vi "img test 4.vi"() -> ()   [LabVIEW 2009]
uses:
  <vilib>/vision/NI_Vision_Development_Module.lvlib
panel:
  in  "Number of Erosion":i32=2
  in  "Number of iterations (1) 3":i32=1
  in  "Structuring Element 3":i32[][](array[numeric])=[[1, 0, 0, 0, 0], [0, 0, 0, 0, 0], [0, 0, 0, 0, 0], [0, 0, 0, 0, 0], [0, 0, 0, 0, 1]]
  in  "Operation 3":T1(ring)=enum."Erode"
  out "appended array":cluster{"Numeric":dbl, "Numeric":dbl}[](array[cluster])
  out "Image 5":T2(plugin-control)
  in  "Number of iterations (1) 2":i32=1
  in  "Structuring Element 2":i32[][](array[numeric])=[[1, 0, 0, 0, 0], [0, 0, 0, 0, 0], [0, 0, 0, 0, 0], [0, 0, 0, 0, 0], [0, 0, 0, 0, 1]]
  in  "Operation 2":T1(ring)=enum."Erode"
  in  "Range 2":cluster{"Lower value":sgl, "Upper value":sgl}={"Lower value"=128.0, "Upper value"=255.0} {"Upper value" format="%.2f"; "Lower value" format="%.2f"}
  out "Image":T2(plugin-control)
  in  "stop":bool
  out "Image 2":T2(plugin-control)
  in  "frame diff":i32
  in  "startign rame":i32
  in  "AVI Path":path=path "C:/Users/Kokum Weeratunga/Desktop/ChongWei vs LinDan (japan open 2010).avi"
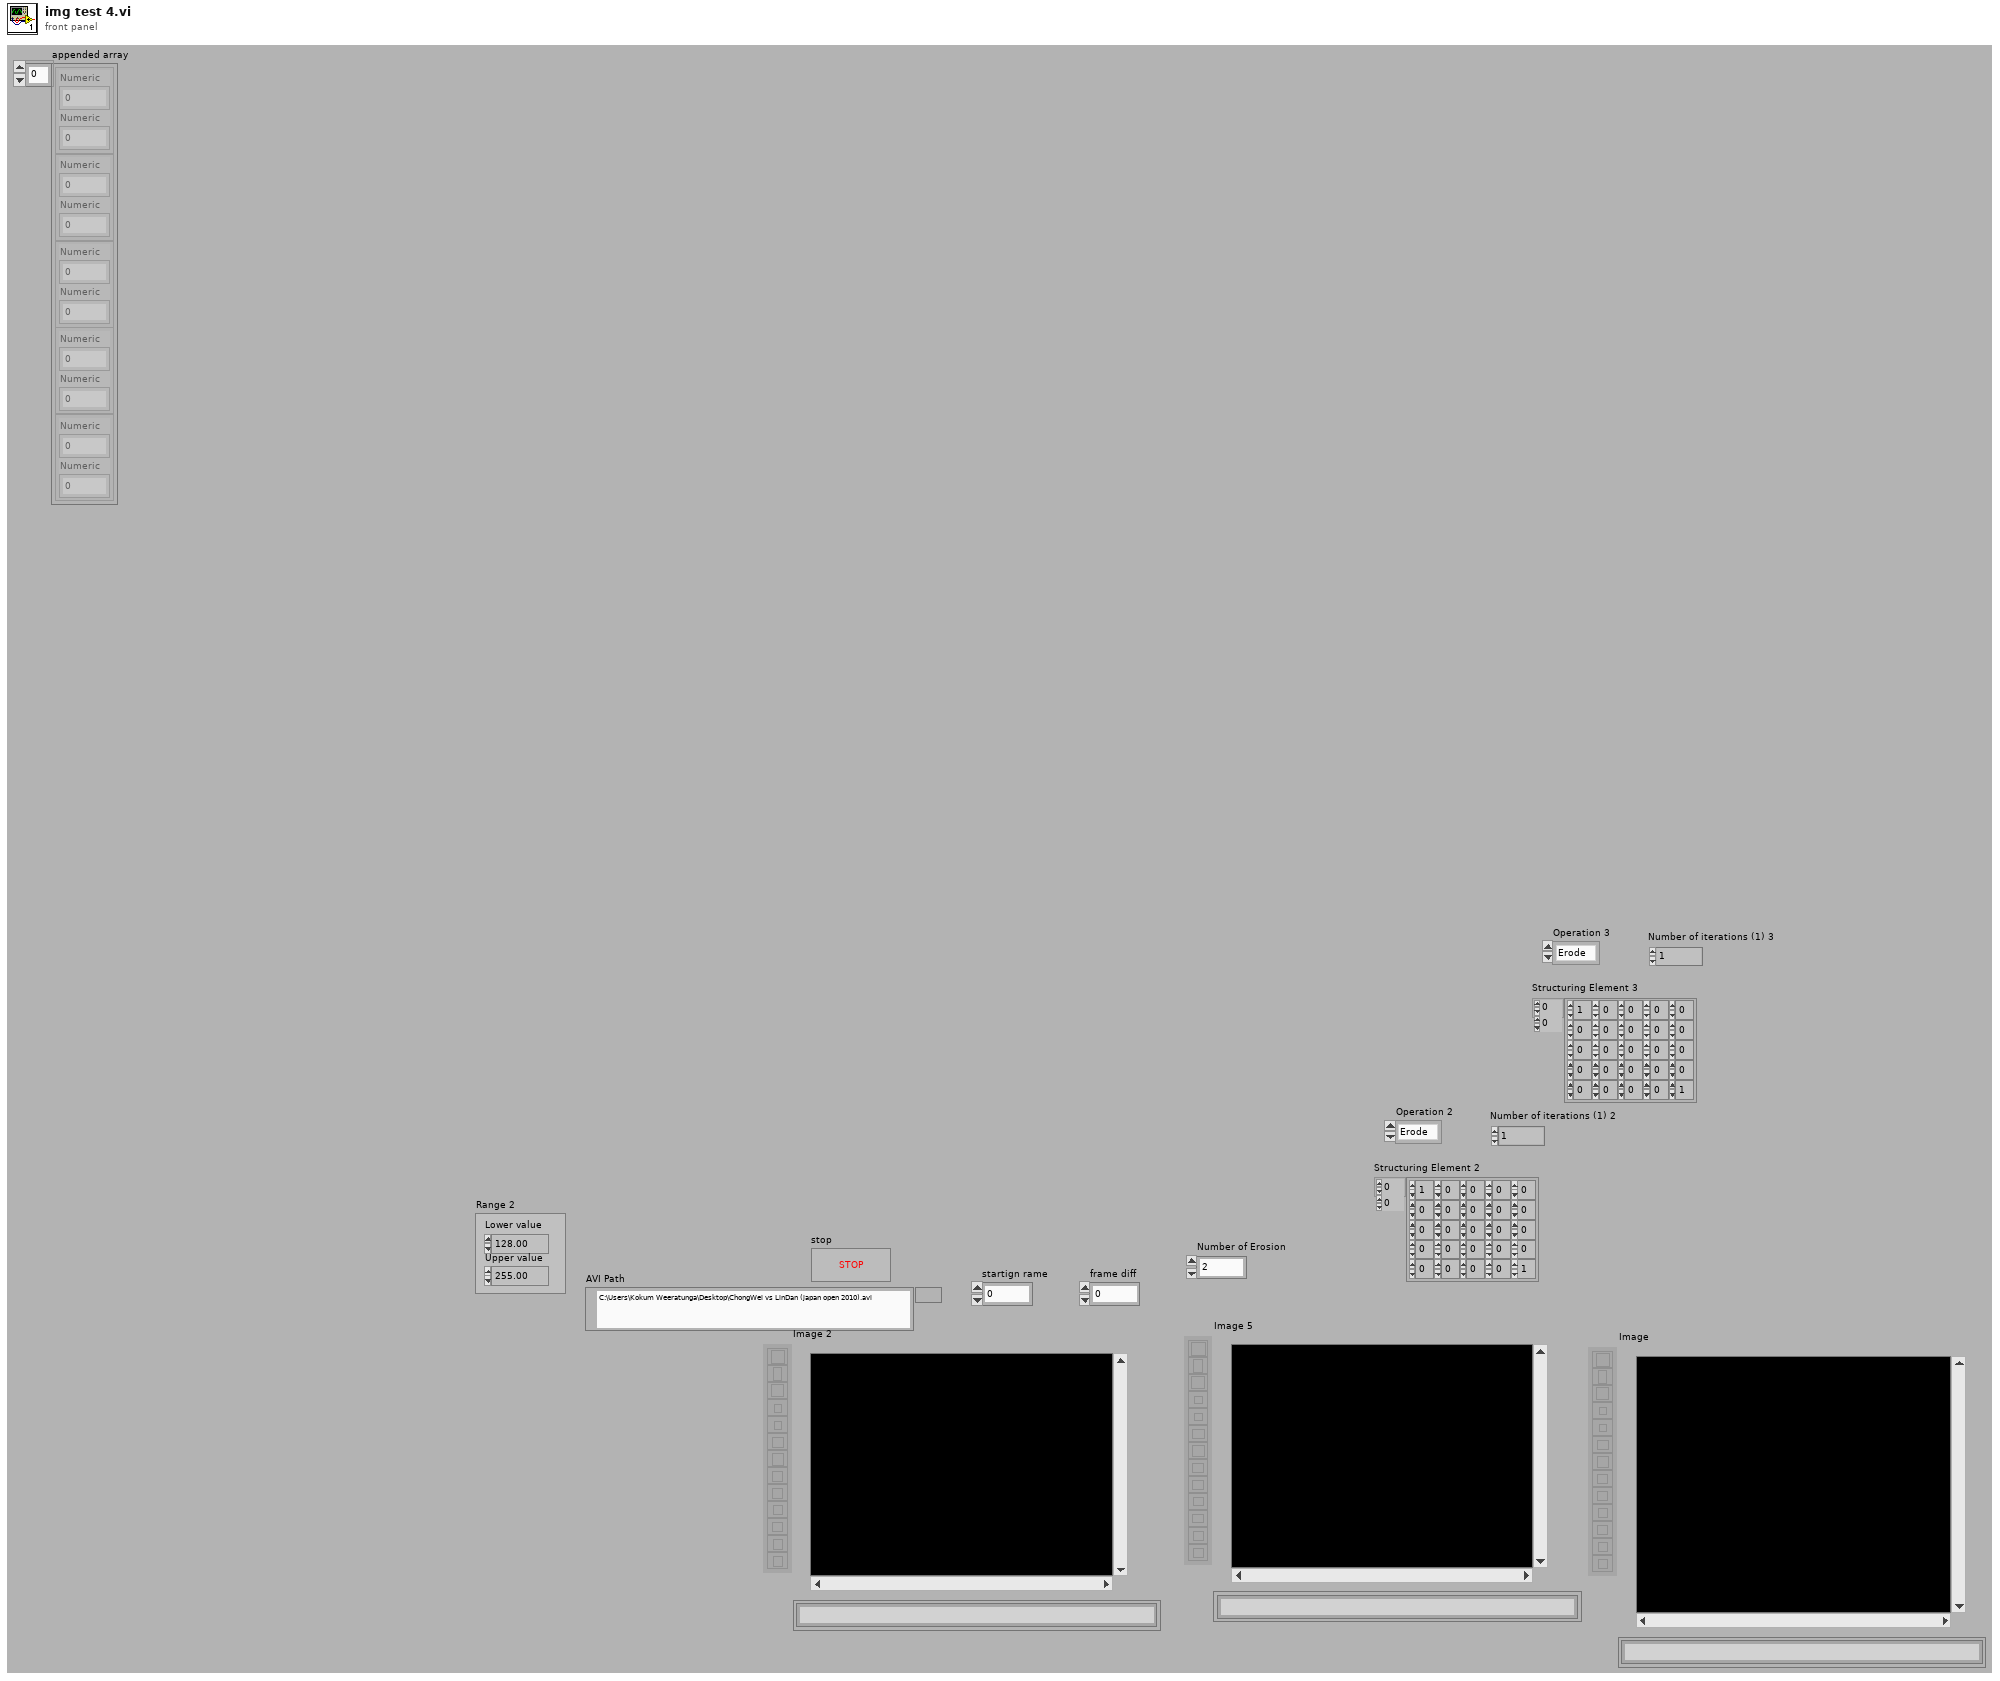
[diagram p1: front panel]
types:
  T1 = enum32{"AutoM", "Close", "Dilate", "Erode", "Gradient", "Gradient in", "Gradient out", "HitMiss", "Open", "PClose", "POpen", "Thick", "Thin"}
  T2 = typedef "IMAQ Image.ctl" = refnum<image>
  T3 = typedef "Image Type" = u32
  T4 = typedef "AviRefnum.ctl" = refnum<k1>
  T5 = typedef "Particle Parameters" = i32
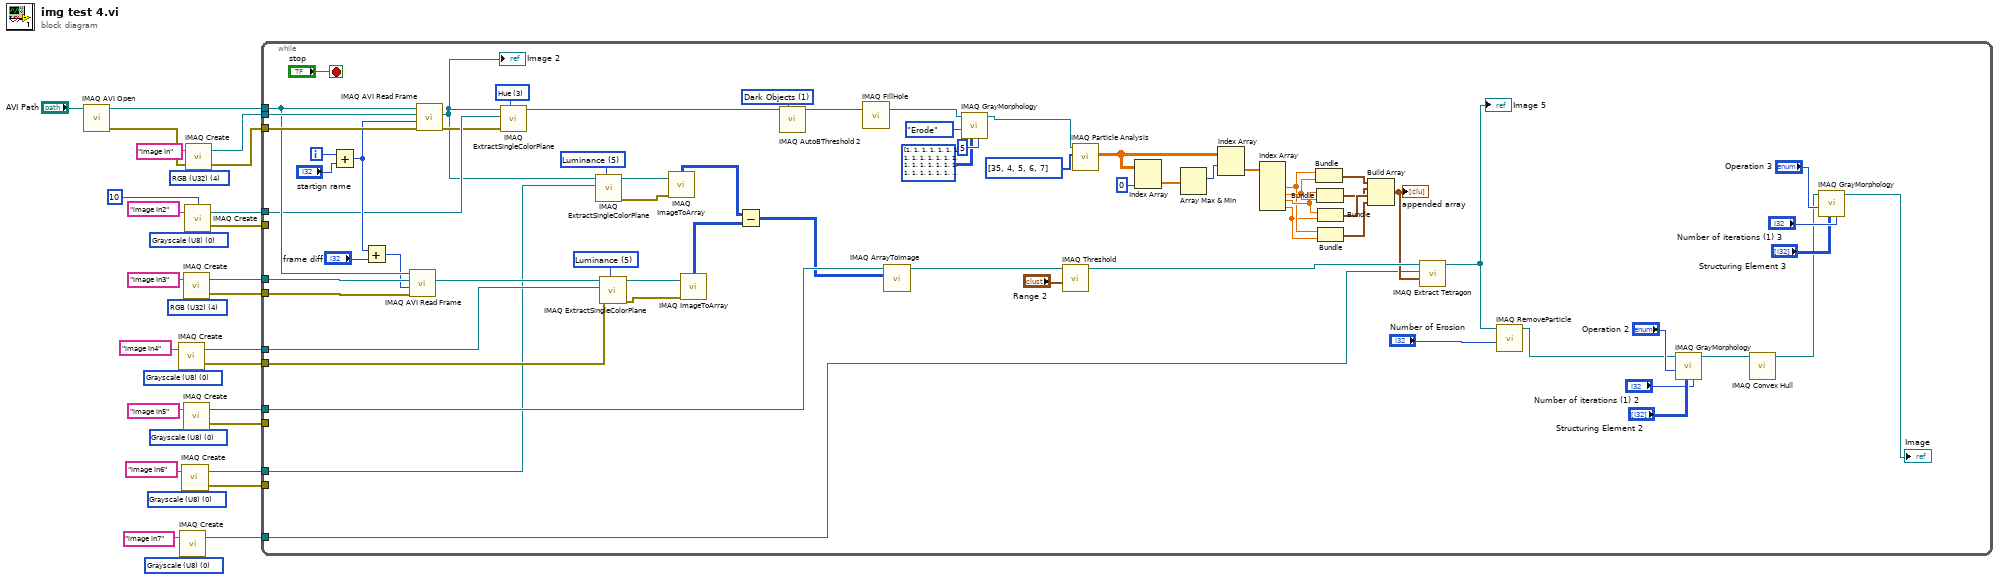
[diagram p0: block diagram]
diagram:
  w3 = T3 0 items=["Grayscale (U8)", "Grayscale (I16)", "Grayscale (SGL)", "Complex (CSG)", "RGB (U32)", "HSL (U32)", "RGB (U64)", "Grayscale (U16)"] ("Image Type")
  w7 = T3 0 items=["Grayscale (U8)", "Grayscale (I16)", "Grayscale (SGL)", "Complex (CSG)", "RGB (U32)", "HSL (U32)", "RGB (U64)", "Grayscale (U16)"] ("Image Type")
  w18 = T3 0 items=["Grayscale (U8)", "Grayscale (I16)", "Grayscale (SGL)", "Complex (CSG)", "RGB (U32)", "HSL (U32)", "RGB (U64)", "Grayscale (U16)"] ("Image Type")
  w16 = T3 4 items=["Grayscale (U8)", "Grayscale (I16)", "Grayscale (SGL)", "Complex (CSG)", "RGB (U32)", "HSL (U32)", "RGB (U64)", "Grayscale (U16)"] ("Image Type")
  w20 = T3 0 items=["Grayscale (U8)", "Grayscale (I16)", "Grayscale (SGL)", "Complex (CSG)", "RGB (U32)", "HSL (U32)", "RGB (U64)", "Grayscale (U16)"] ("Image Type")
  w23 = T3 0 items=["Grayscale (U8)", "Grayscale (I16)", "Grayscale (SGL)", "Complex (CSG)", "RGB (U32)", "HSL (U32)", "RGB (U64)", "Grayscale (U16)"] ("Image Type")
  w26 = T3 4 items=["Grayscale (U8)", "Grayscale (I16)", "Grayscale (SGL)", "Complex (CSG)", "RGB (U32)", "HSL (U32)", "RGB (U64)", "Grayscale (U16)"] ("Image Type")
  n1 = call "IMAQ AVI Open"("AVI Path"="AVI Path") -> ("error out"=w30:errorcluster, "Avi Refnum"=w25:T4)  [unwired: 9 in]
  n2 = call "IMAQ Create"("Image Name"="image in4", "Image Type"=w18) -> ("New Image"=w12:T2, "error out"=w11:errorcluster)  [unwired: 3 in]
  n3 = call "IMAQ Create"("Image Name"="image in7", "Image Type"=w3) -> ("New Image"=w2:T2)  [unwired: 3 in, 1 out]
  n4 = call "IMAQ Create"("Image Name"="image in6", "Image Type"=w7) -> ("New Image"=w6:T2, "error out"=w5:errorcluster)  [unwired: 3 in]
  n5 = call "IMAQ Create"("Image Name"="image in3", "Image Type"=w16) -> ("New Image"=w14:T2, "error out"=w13:errorcluster)  [unwired: 3 in]
  n6 = call "IMAQ Create"("Image Name"="image in5", "Image Type"=w20) -> ("New Image"=w10:T2, "error out"=w9:errorcluster)  [unwired: 3 in]
  n7 = call "IMAQ Create"("Border Size"=10, "Image Name"="image in2", "Image Type"=w23) -> ("New Image"=w22:T2, "error out"=w21:errorcluster)  [unwired: 2 in]
  n8 = call "IMAQ Create"("Image Name"="image in", "Image Type"=w26, "error in (no error)"=w30) -> ("New Image"=w27:T2, "error out"=w28:errorcluster)  [unwired: 2 in]
  n9 = while {
    tunnel: w28 -> [w99]
    tunnel: w27 -> [w98]
    tunnel: w25 -> [w96]
    tunnel: w22 -> [w87]
    tunnel: w21 -> [_]
    tunnel: w14 -> [w95]
    tunnel: w13 -> [w94]
    tunnel: w12 -> [w84]
    tunnel: w11 -> [w83]
    tunnel: w10 -> [w88]
    tunnel: w9 -> [_]
    tunnel: w6 -> [w46]
    tunnel: w5 -> [_]
    tunnel: w2 -> [w32]
    i -> [w92]
    stop <- "stop" stop-if-true
    w47 = 5 items=["Red", "Green", "Blue", "Hue", "Saturation", "Luminance", "Value", "Intensity"] ("Color Plane")
    w60 = T5[] [35, 4, 5, 6, 7] items=["Center of Mass X", "Center of Mass Y", "First Pixel X", "First Pixel Y", "Bounding Rect Left", "Bounding Rect Top", "Bounding Rect Right", "Bounding Rect Bottom", "Max Feret Diameter Start X", "Max Feret Diameter Start Y", "Max Feret Diameter End X", "Max Feret Diameter End Y", "Max Horiz. Segment Length Left", "Max Horiz. Segment Length Right", "Max Horiz. Segment Length Row", "-", "Bounding Rect Width", "Bounding Rect Height", "Bounding Rect Diagonal", "Perimeter", "Convex Hull Perimeter", "Holes' Perimeter", "Max Feret Diameter", "Equivalent Ellipse Major Axis", "Equivalent Ellipse Minor Axis", "Equivalent Ellipse Minor Axis (Feret)", "Equivalent Rect Long Side", "Equivalent Rect Short Side", "Equivalent Rect Diagonal", "Equivalent Rect Short Side (Feret)", "Average Horiz. Segment Length", "Average Vert. Segment Length", "Hydraulic Radius", "Waddel Disk Diameter", "-", "Area", "Holes' Area", "Particle & Holes' Area", "Convex Hull Area", "Image Area", "-", "Number of Holes", "Number of Horiz. Segments", "Number of Vert. Segments", "-", "Orientation", "Max Feret Diameter Orientation", "-", "% Area/Image Area", "% Area/(Particle & Holes' Area)", "Ratio of Equivalent Ellipse Axes", "Ratio of Equivalent Rect Sides", "-", "Elongation Factor", "Compactness Factor", "Heywood Circularity Factor", "Type Factor", "-", "Sum X", "Sum Y", "Sum XX", "Sum XY", "Sum YY", "Sum XXX", "Sum XXY", "Sum XYY", "Sum YYY", "-", "Moment of Inertia XX", "Moment of Inertia XY", "Moment of Inertia YY", "Moment of Inertia XXX", "Moment of Inertia XXY", "Moment of Inertia XYY", "Moment of Inertia YYY", "Norm. Moment of Inertia XX", "Norm. Moment of Inertia XY", "Norm. Moment of Inertia YY", "Norm. Moment of Inertia XXX", "Norm. Moment of Inertia XXY", "Norm. Moment of Inertia XYY", "Norm. Moment of Inertia YYY", "Hu Moment 1", "Hu Moment 2", "Hu Moment 3", "Hu Moment 4", "Hu Moment 5", "Hu Moment 6", "Hu Moment 7"] ("Pixel Measurements")
    w54 = u32 1 items=["Bright Objects", "Dark Objects"] ("Look For (Bright Objects)")
    w82 = 5 items=["Red", "Green", "Blue", "Hue", "Saturation", "Luminance", "Value", "Intensity"] ("Color Plane")
    w85 = 3 items=["Red", "Green", "Blue", "Hue", "Saturation", "Luminance", "Value", "Intensity"] ("Color Plane")
    n10 = Add(x=w92, y="startign rame") -> (x+y=w90:i32)
    n11 = Add(x=w90, y="frame diff") -> (x+y=w93:i32)
    n12 = call "IMAQ AVI Read Frame"("error in (no error)"=w94, "Frame Number"=w93, "Image"=w95, "Avi Refnum"=w96) -> ("Image Out"=w81:T2)  [unwired: 4 in, 3 out]
    n13 = call "IMAQ AVI Read Frame"("error in (no error)"=w99, "Frame Number"=w90, "Image"=w98, "Avi Refnum"=w96) -> ("error out"=w86:errorcluster, "Image Out"=w33:T2)  [unwired: 4 in, 2 out]
    "Image 2" <- w33
    n14 = call "IMAQ ExtractSingleColorPlane"("Color Plane"=w85, "error in (no error)"=w86, "Image Dst"=w87, "Image Src"=w33) -> ("Image Dst Out"=w34:T2)  [unwired: 6 in, 1 out]
    n15 = call "IMAQ ExtractSingleColorPlane"("Color Plane"=w47, "Image Dst"=w46, "Image Src"=w33) -> ("error out"=w49:errorcluster, "Image Dst Out"=w48:T2)  [unwired: 7 in]
    n16 = call "IMAQ ExtractSingleColorPlane"("Color Plane"=w82, "error in (no error)"=w83, "Image Dst"=w84, "Image Src"=w81) -> ("error out"=w45:errorcluster, "Image Dst Out"=w71:T2)  [unwired: 6 in]
    n17 = call "IMAQ ImageToArray"("error in (no error)"=w49, "Image"=w48) -> ("Image Pixels (U8)"=w79:u8[][])  [unwired: 2 in, 4 out]
    n18 = call "IMAQ ImageToArray"("error in (no error)"=w45, "Image"=w71) -> ("Image Pixels (U8)"=w80:u8[][])  [unwired: 2 in, 4 out]
    n19 = Subtract(x=w79, y=w80) -> (x-y=w78:u8[][])
    n20 = call "IMAQ AutoBThreshold 2"("Image Src"=w34, "Look For (Bright Objects)"=w54) -> ("Image Dst Out"=w55:T2)  [unwired: 11 in, 2 out]
    n21 = call "IMAQ FillHole"("Image Src"=w55) -> ("Image Dst Out"=w58:T2)  [unwired: 5 in, 1 out]
    n22 = call "IMAQ ArrayToImage"("Image Pixels (U8)"=w78, "Image"=w88) -> ("Image Out"=w76:T2)  [unwired: 8 in, 1 out]
    n23 = call "IMAQ GrayMorphology"("Number of iterations (1)"=5, "Structuring Element"=i32[][] [[1, 1, 1, 1, 1, 1, 1, 1, 1, 1], [1, 1, 1, 1, 1, 1, 1, 1, 1, 1], [1, 1, 1, 1, 1, 1, 1, 1, 1, 1], [1, 1, 1, 1, 1, 1, 1, 1, 1, 1], [1, 1, 1, 1, 1, 1, 1, 1, 1, 1], [1, 1, 1, 1, 1, 1, 1, 1, 1, 1], [1, 1, 1, 1, 1, 1, 1, 1, 1, 1]], "Operation"=T1."Erode", "Image Src"=w58) -> ("Image Dst Out"=w36:T2)  [unwired: 6 in, 1 out]
    n24 = call "IMAQ Threshold"("Range"="Range 2", "Image Src"=w76) -> ("Image Dst Out"=w50:T2)  [unwired: 8 in, 1 out]
    n25 = call "IMAQ Particle Analysis"("Pixel Measurements"=w60, "Image"=w36) -> ("Particle Measurements (Pixels)"=w63:dbl[][])  [unwired: 4 in, 5 out]
    n26 = Index Array(array=w63, index (col)=0 ("disabled index (col)")) -> (element=w62:dbl[])  [unwired: 1 in]
    n27 = Array Max & Min(array=w62) -> (max index (indices)=w64:i32)  [unwired: 3 out]
    n28 = Index Array(array=w63, index (row)=w64) -> (element=w65:dbl[])  [unwired: 1 in]
    n29 = Index Array(array=w65) -> (element #2=w53:dbl, element #3=w70:dbl, element #4=w69:dbl, element #5=w52:dbl)  [unwired: 5 in, 1 out]
    n30 = Bundle("Numeric"=w53, "Numeric"=w70) -> (w66:cluster{"Numeric":dbl, "Numeric":dbl})  [unwired: 1 in]
    n31 = Bundle("Numeric"=w69, "Numeric"=w70) -> (w67:cluster{"Numeric":dbl, "Numeric":dbl})  [unwired: 1 in]
    n32 = Bundle("Numeric"=w69, "Numeric"=w52) -> (w68:cluster{"Numeric":dbl, "Numeric":dbl})  [unwired: 1 in]
    n33 = Bundle("Numeric"=w53, "Numeric"=w52) -> (w51:cluster{"Numeric":dbl, "Numeric":dbl})  [unwired: 1 in]
    n34 = Build Array(w66, w67, w68, w51) -> (w35:cluster{"Numeric":dbl, "Numeric":dbl}[])
    "appended array" <- w35
    n35 = call-poly "IMAQ Extract Tetragon"("Tetragon"=w35, "Image Dst"=w32, "Image Src"=w50) -> ("Image Dst Out"=w39:T2)  [unwired: 7 in, 1 out]
    "Image 5" <- w39
    n36 = call "IMAQ RemoveParticle"("Number of Erosion"="Number of Erosion", "Image Src"=w39) -> ("Image Dst Out"=w38:T2)  [unwired: 8 in, 1 out]
    n37 = call "IMAQ GrayMorphology"("Number of iterations (1)"="Number of iterations (1) 2", "Structuring Element"="Structuring Element 2", "Operation"="Operation 2", "Image Src"=w38) -> ("Image Dst Out"=w72:T2)  [unwired: 6 in, 1 out]
    n38 = call "IMAQ Convex Hull"("Image Src"=w72) -> ("Image Dst Out"=w40:T2)  [unwired: 9 in, 1 out]
    n39 = call "IMAQ GrayMorphology"("Number of iterations (1)"="Number of iterations (1) 3", "Structuring Element"="Structuring Element 3", "Operation"="Operation 3", "Image Src"=w40) -> ("Image Dst Out"=→"Image":T2)  [unwired: 6 in, 1 out]
  }
